vi "tearDown.vi"(8 "error in (no error)":errorcluster, 11 "reference in":refnum<class "BufferedArray_Functional.lvclass">) -> (0 "error out":errorcluster, 3 "reference out":refnum<class "BufferedArray_Functional.lvclass">)   [LabVIEW 2009, in "BufferedArray_Functional.lvclass"]
doc: "tearDown runs after the test method has completed. Use this method to clean up any operations or references that were opened by setUp or the test method. Unit tests should be independent of other unit tests so this VI should ensure that the next test can run in a 'clean' test environment."
uses:
  BufferedArray_Functional.lvclass
  BufferedArray_Functional.lvclass/BufferedArray_Functional.ctl
  source/Lists/List/List.lvclass
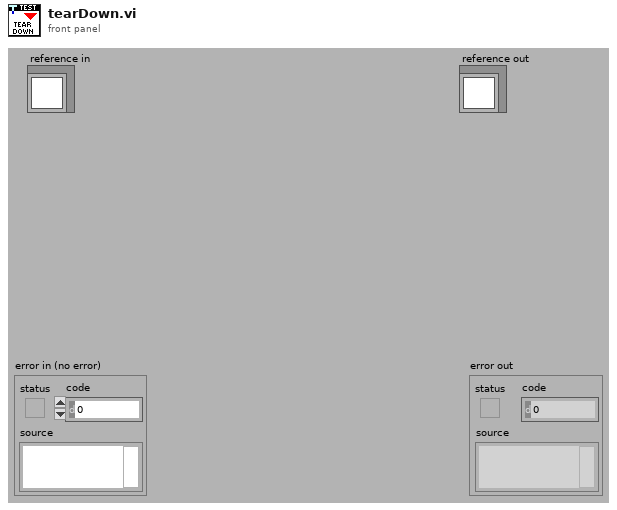
[diagram p1: front panel]
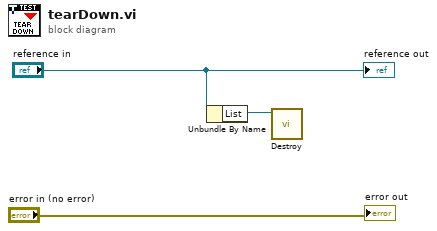
[diagram p0: block diagram]
diagram:
  n1 = Unbundle By Name("reference in") -> ("List"=w1:refnum<class "List.lvclass">)
  n2 = call-dynamic "Destroy.vi"("List in"=w1) -> ()  [unwired: 10 in, 1 out]
  "error out" <- "error in (no error)"
  "reference out" <- "reference in"
